vi "Read Job Build Info.vi"(8 "error in (no error)":errorcluster, 11 "Build Job in":refnum<class "Build Job.lvclass">) -> (0 "error out":errorcluster, 2 "Job Build Info":T1, 3 "Build Job out":refnum<class "Build Job.lvclass">)   [LabVIEW 2014, in "Build Job.lvclass"]
uses:
  Build Job.lvclass
  Controls/Job Build Info - STYP.ctl
  Build Job.lvclass/Build Job.ctl
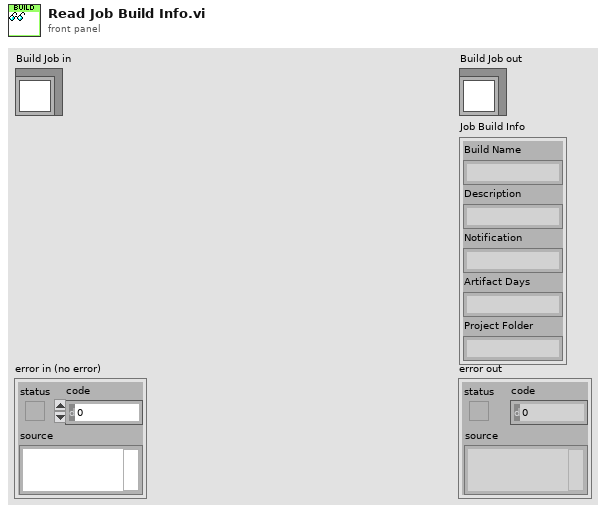
[diagram p1: front panel]
types:
  T1 = typedef "Job Build Info - STYP.ctl" = cluster{"Build Name":string, "Description":string, "Notification":string, "Artifact Days":string, "Project Folder":string}
  T2 = cluster{"[0]":string, "[1]":string, "[2]":string, "[3]":string, "[4]":string}
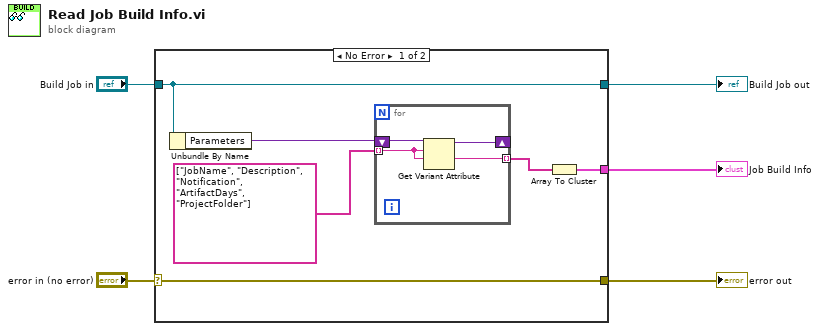
[diagram p0: block diagram]
diagram:
  n1 = case shown="No Error" "error in (no error)" {
    selector: "error in (no error)" -> [w11 w16]
    tunnel: [w11 w16] -> w4
    tunnel: [w10 w17] -> w2
    tunnel: "Build Job in" -> [w10 w17]
    tunnel: [w6 _] -> w1
    frame No Error {
      n2 = Unbundle By Name(w10) -> ("Parameters"=w9:variant)
      n3 = for {
        shift-right: [w14] -> _
        shift-left: w9 -> [w15]
        tunnel: string[] ["JobName", "Description", "Notification", "ArtifactDays", "ProjectFolder"] -> [w13] mode=indexing
        tunnel: [w12] -> w7 mode=indexing
        n4 = Get Variant Attribute(Variant=w15, name=w13, default value (empty Variant)=w13) -> (duplicate Variant=w14:variant, value=w12:string)  [unwired: 1 in, 2 out]
      }
      n5 = Array To Cluster(array=w7) -> (cluster=w6:T2)
    }
    frame Error {
    }
  }
  "error out" <- w4
  "Build Job out" <- w2
  "Job Build Info" <- w1
